vi "5.7.4-UDP-Forbrain_to_OCU-Server.vi"() -> ()   [LabVIEW 2010]
doc: "Creates a named service and listens on the first available port. Whenever a client connects to the service, it responds with a message containing joystick data. The VI can be stopped using the STOP button."
uses:
  6-OCU Neurons/CommonIndicators.ctl
  5.0-Global.vi
panel:
  out "5.7.2 Main Indicators":T1={"Speed"=0.0, " Heading"={0.0, 34.390870865624734}, "MissionTime"=0.0, "Battery"=0.0, "MAP"=FALSE, "LIDAR"=FALSE, "ManualMissionMap"=bytes[0], "ManualModeLIDAR"=bytes[0], "ManualModeStop"=FALSE, "How?"=FALSE, "Where?"=FALSE, "What?"=FALSE, "ActManual"=FALSE, "CollisionLight "=FALSE, "Ready"=FALSE} {"Battery" scale=16.0..24.0; "MissionTime" scale=0.0..10.0; "Heading" scale=180.0..-180.0; "Speed" scale=0.0..4.0}
  out "data out":string
  out "error out":errorcluster
  in  "error in":errorcluster
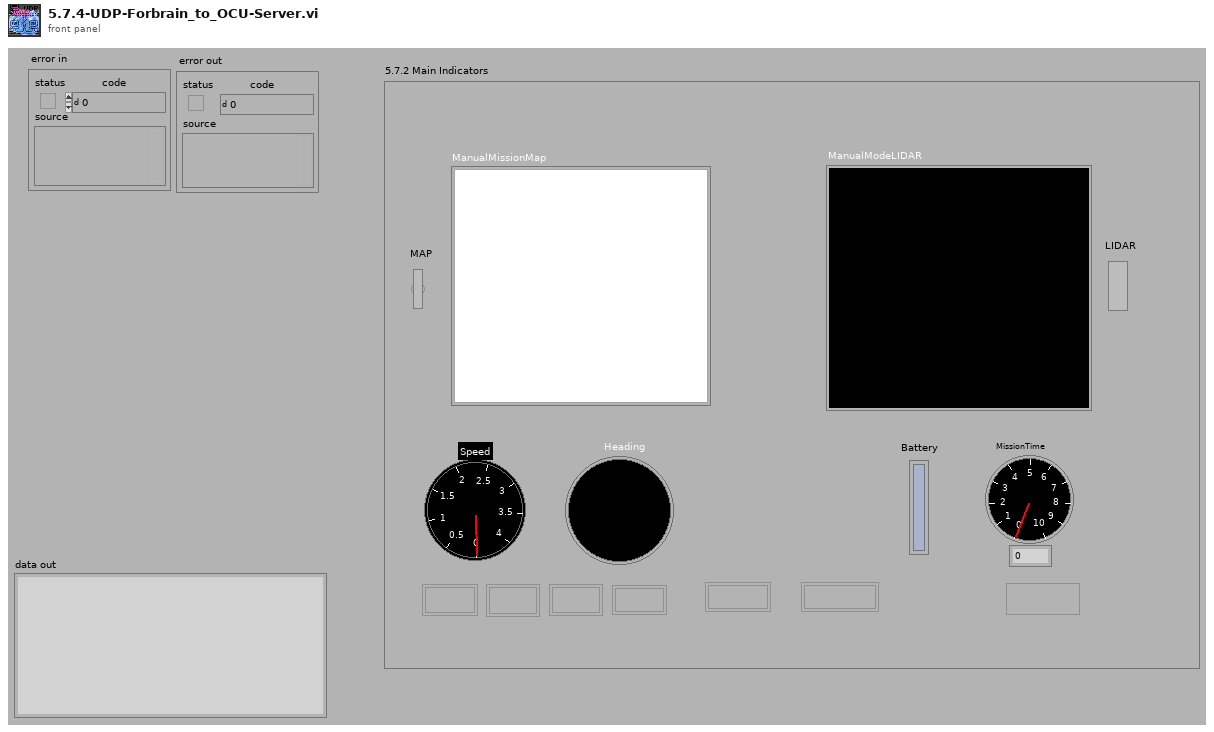
[diagram p1: front panel]
types:
  T1 = typedef "CommonIndicators.ctl" = cluster{"Speed":dbl, " Heading":cluster{dbl, dbl}, "MissionTime":dbl, "Battery":dbl, "MAP":bool, "LIDAR":bool, "ManualMissionMap":picture, "ManualModeLIDAR":picture, "ManualModeStop":bool, "How?":bool, "Where?":bool, "What?":bool, "ActManual":bool, "CollisionLight ":bool, "Ready":bool}
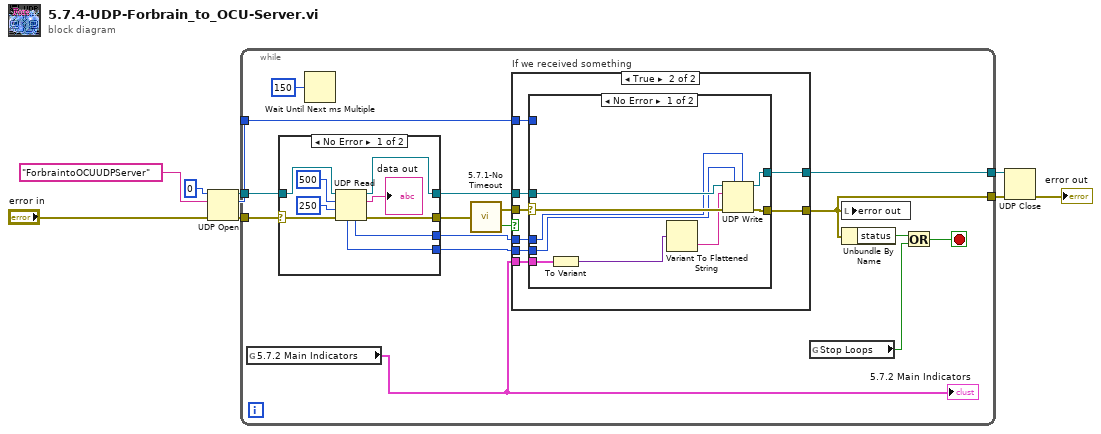
[diagram p0: block diagram]
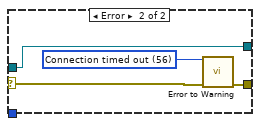
[diagram p3: hidden frame]
diagram:
  n1 = UDP Open(8:"error in", 10:"ForbraintoOCUUDPServer", 11:0) -> (port=w7:refnum<k16>, 0:w6:errorcluster, 2:w2:u16)  [unwired: 2 in]
  n2 = while {
    tunnel: [w14] -> w4
    tunnel: w7 -> [w25]
    tunnel: w6 -> [w22]
    tunnel: [w23] -> w5
    tunnel: w2 -> [w19]
    stop <- w17 stop-if-true
    n3 = global read "5.0-Global.vi" "5.7.2 Main Indicators"() -> (w11:T1)
    "5.7.2 Main Indicators" <- w11
    n4 = case shown="No Error" w22 {
      selector: w22 -> [w55 w58]
      tunnel: w25 -> [w57 w59]
      tunnel: [w54 w59] -> w24
      tunnel: [w53 w58] -> w13
      tunnel: [w51 _] -> w20
      tunnel: [w52 _] -> w21
      frame No Error {
        n5 = UDP Read(connection ID=w57, max size (548)=500, timeout ms (25000)=250, 8:w55) -> (data out=→"data out":string, error out=w53:errorcluster, 3:w54:refnum<k16>, 4:w51:u16, 6:w52:u32)
      }
      frame Error {
      }
    }
    n6 = Wait Until Next ms Multiple(millisecond multiple=u32 150) -> ()  [unwired: 1 out]
    n7 = call "5.7.1-No Timeout.vi"("error in (no error)"=w13) -> ("No Timeout"=w15:bool, "error out"=w16:errorcluster)
    n8 = case "If we received something" shown="True" w15 {
      tunnel: w24 -> [w26 w35]
      tunnel: [w26 w34] -> w23
      tunnel: w21 -> [_ w33]
      tunnel: w20 -> [_ w32]
      tunnel: w19 -> [_ w31]
      tunnel: [w27 w30] -> w14
      tunnel: w16 -> [w27 w29]
      tunnel: w11 -> [_ w28]
      frame False {
      }
      frame True {
        n9 = case shown="No Error" w29 {
          selector: w29 -> [w44 w46]
          tunnel: w35 -> [w41 w48]
          tunnel: [w43 w45] -> w30
          tunnel: [w42 w48] -> w34
          tunnel: w33 -> [w39 _]
          tunnel: w32 -> [w40 _]
          tunnel: w31 -> [_ _]
          tunnel: w28 -> [w36 _]
          frame No Error {
            n10 = To Variant(anything=w36) -> (Variant=w38:variant)
            n11 = Variant To Flattened String(Variant=w38) -> (data string=w37:string)  [unwired: 1 out]
            n12 = UDP Write(address=w39, port or service name=w40, connection ID=w41, data in=w37, 8:w44) -> (error out=w43:errorcluster, 3:w42:refnum<k16>)  [unwired: 1 in]
          }
          frame Error {
            w47 = 56 items=["No Error", "Argument Error", "Memory Full", "Out of Zone", "End of File", "File Already Open", "Generic File IO Error", "File Not Found", "File Permission Error", "Disk Full", "Duplicate Path", "Too Many Files Open", "Not Enabled", "Resource File Not Found", "Cannot Add Resource", "Resource Not Found", "Image Not Found", "Image Memory Error", "Pen Does Not Exist", "Config Bad Type", "Config Token Not Found", "Config Parse Error", "Config Memory Error", "Bad External Code Format", "Bad External Code Offset", "External Code Not Present", "Null Window", "Destroy Window Mixup", "Null Menu", "Print Aborted", "Bad Print Record", "Print Driver Error", "Windows Error During Print", "Memory Error During Print", "Print Dialog Error", "Generic Print Error", "Invalid Device Refnum", "Device Not Found", "Device Parameter Error", "Device Unit Error", "Can't Open Device", "Device Call Aborted", "Generic Error", "Cancelled By User", "Object ID Too Low", "Object ID Too High", "Object Not In Heap", "Unknown Heap", "Bad DefProc ID", "DefProc Not In Table", "Message Out Of Range", "Null Method", "Unknown Message", "Manager Call Not Supported", "Bad address", "Connection In progress", "Connection timed out", "Connection is already in progress", "Network attribute not supported", "Network error", "Address in use", "System out of memory", "Connection aborted", "Connection refused", "Connection is not connected", "Connection is already connected", "Connection closed", "Initialize error (interapplication manager)", "Bad occurrence", "Wait on unbound occurrence handler", "Occurrence queue overflow", "Bad path", "Semaphore not signaled", "Unrecognized type (interapplication manager)"] ("1st Error to Convert")
            n13 = call <vilib>:"Error to Warning.vi"("1st Error to Convert"=w47, "error in"=w46) -> ("warning out"=w45:errorcluster)  [unwired: 13 in]
          }
        }
      }
    }
    n14 = global read "5.0-Global.vi" "Stop Loops"() -> (w12:bool)
    n15 = local write "error out"(w14) -> ()
    n16 = Unbundle By Name(w14) -> ("status"=w18:bool)
    n17 = Or(x=w18, y=w12) -> (x .or. y?=w17:bool)
  }
  n18 = UDP Close(connection ID=w5, 8:w4) -> (error out=→"error out":errorcluster)  [unwired: 1 out]
